vi "Set Decimation.vi"(8 "error in (no error)":errorcluster, 9 "Min decimation":u32=4, 10 "Decimation":u32, 11 "RP Instrument in":refnum<class "RP Instrument.lvclass">) -> (0 "error out":errorcluster, 3 "RP Instrument out":refnum<class "RP Instrument.lvclass">)   [LabVIEW 2024, in "RP Instrument.lvclass"]
uses:
  RP Instrument.lvclass
  RP Instrument.lvclass/RP Instrument.ctl
  RP Config Offsets.ctl
  RP Command.ctl
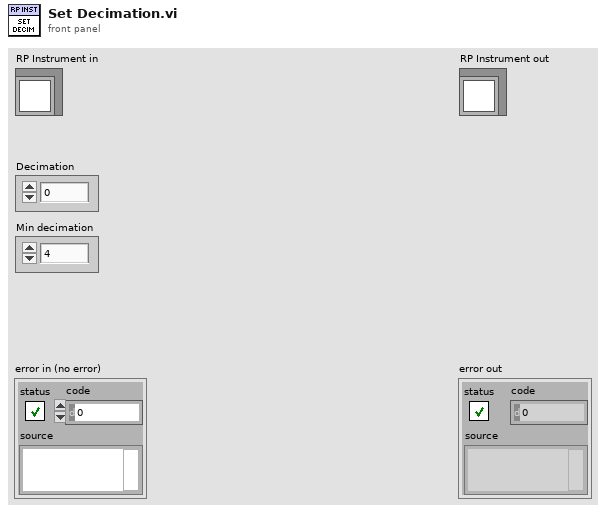
[diagram p1: front panel]
types:
  T1 = typedef "RP Command.ctl" = enum16{"Reset", "Read IDN", "Stop server", "Get status", "Get temperature", "Connect client", "Arm", "Software trigger", "Get whole buffer", "Get chunk", "System call", "Get config", "Set config", "Recieve data", "Recieve Calibartion", "Transmit data"}
  T2 = typedef "RP Config Offsets.ctl" = u16
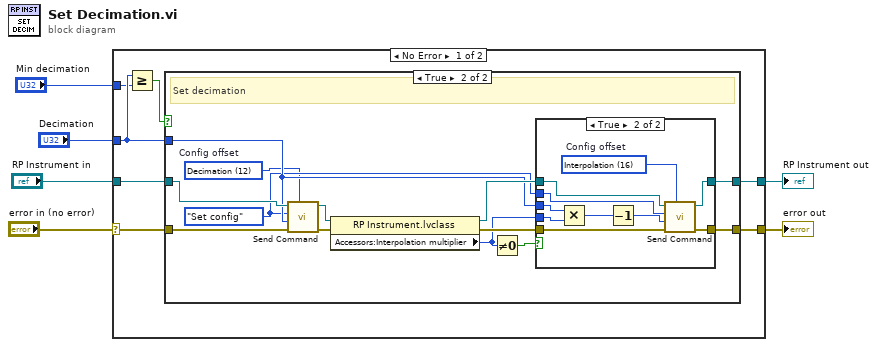
[diagram p0: block diagram]
diagram:
  n1 = case shown="No Error" "error in (no error)" {
    selector: "error in (no error)" -> [w13 w42]
    tunnel: [w12 w42] -> w5
    tunnel: [w8 w41] -> w3
    tunnel: "RP Instrument in" -> [w7 w41]
    tunnel: "Decimation" -> [w10 _]
    tunnel: "Min decimation" -> [w9 _]
    frame No Error {
      n2 = Greater Or Equal?(x=w10, y=w9) -> (x >= y?=w11:bool)
      n3 = case shown="True" w11 {
        tunnel: w13 -> [w15 w27]
        tunnel: [w15 w22] -> w12
        tunnel: w10 -> [_ w19]
        tunnel: w7 -> [w14 w28]
        tunnel: [w14 w20] -> w8
        frame False {
        }
        frame True {
          w17 = RP_Command."Set config" ("Command number")
          w16 = T2 12 items=["Config flags"=0, "Record length"=4, "Frequency 0"=8, "Decimation"=12, "Interpolation"=16, "DDS delay"=28, "Fequency 1"=56, "Amplitude 1"=60]  # Config offset
          # "Set decimation"
          n4 = call-dynamic "Send Command.vi"("Config offset"=w16, "error in (no error)"=w27, "Command payload"=w19, "Command number"=w17, "RP Instrument in"=w28) -> ("error out"=w26:errorcluster, "RP Instrument out"=w25:refnum<class "RP Instrument.lvclass">)  [unwired: 5 in]
          n5 = property class="RP Instrument.lvclass"(reference=w25, error in=w26) -> (reference out=w21:refnum<class "RP Instrument.lvclass">, error out=w23:errorcluster, "Accessors:Interpolation multiplier"=w18:u32)
          n6 = Not Equal To 0?(x=w18) -> (x != 0?=w24:bool)
          n7 = case shown="True" w24 {
            tunnel: w21 -> [w30 w40]
            tunnel: w23 -> [w29 w39]
            tunnel: [w29 w38] -> w22
            tunnel: [w30 w37] -> w20
            tunnel: w19 -> [_ w36]
            tunnel: w18 -> [_ w35]
            tunnel: w17 -> [_ w32]
            frame False {
            }
            frame True {
              w31 = T2 16 items=["Config flags"=0, "Record length"=4, "Frequency 0"=8, "Decimation"=12, "Interpolation"=16, "DDS delay"=28, "Fequency 1"=56, "Amplitude 1"=60]  # Config offset
              n8 = Multiply(x=w36, y=w35) -> (x*y=w34:u32)
              n9 = Decrement(x=w34) -> (x-1=w33:u32)
              n10 = call-dynamic "Send Command.vi"("Config offset"=w31, "error in (no error)"=w39, "Command payload"=w33, "Command number"=w32, "RP Instrument in"=w40) -> ("error out"=w38:errorcluster, "RP Instrument out"=w37:refnum<class "RP Instrument.lvclass">)  [unwired: 5 in]
            }
          }
        }
      }
    }
    frame Error {
    }
  }
  "error out" <- w5
  "RP Instrument out" <- w3
